vi "alarmes.vi"(0 "NXT IN":T1) -> (1 "NXT OUT":T1, 2 "FinalizarPrograma?":bool)   [LabVIEW 2015, in "ExemploFinal.lvrbt"]
uses:
  ExemploFinal.lvrbt
  <vilib>/NXT/Subs/LVHSConnector.ctl
  <vilib>/NXT/LegoClasses/BrickReference/BrickReference.lvclass
  <vilib>/NXT/Dual Mode Library/Waits/Wait_Num.vi
  <vilib>/NXT/Dual Mode Library/Sound/PlayC.vi
  <vilib>/NXT/Dual Mode Library/Sound/PlayB.vi
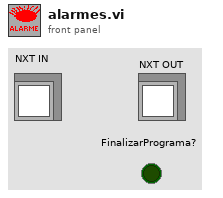
[diagram p1: front panel]
types:
  T1 = typedef "LVHSConnector.ctl" = refnum<class "BrickReference.lvclass">
  T2 = cluster{"TouchOUT":bool, "SomOUT":i32, "LuzOUT":i32, "UltrasomOUT":i32, "BotãoOUT":bool}
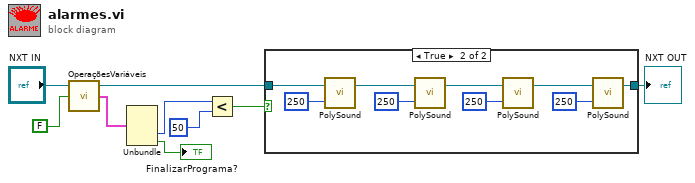
[diagram p0: block diagram]
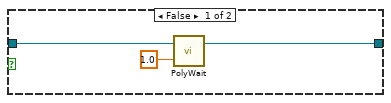
[diagram p2: hidden frame]
diagram:
  n1 = call "OperaçõesVariáveis.vi"("Escrever?"=FALSE, "NXT IN"="NXT IN") -> ("Saídas"=w7:T2, "NXT OUT"=w4:T1)  [unwired: 1 in, 1 out]
  n2 = Unbundle(w7) -> ("UltrasomOUT"=w9:i32, "BotãoOUT"=→"FinalizarPrograma?":bool)  [unwired: 3 out]
  n3 = Less?(x=w9, y=50) -> (x < y?=w2:bool)
  n4 = case shown="True" w2 {
    tunnel: w4 -> [w12 w14]
    tunnel: [w11 w13] -> w6
    frame False {
      n5 = call-poly <vilib>:"PolyWait.vi"("Time (1 sec)"=sgl 1.0, "NXT/EV3"=w12) -> ("NXT/EV3"=w11:T1)  [unwired: 2 in]
    }
    frame True {
      n6 = call-poly <vilib>:"PolySound.vi"("Duration (500 ms)"=u16 250, "NXT/EV3"=w14) -> ("NXT/EV3"=w18:T1)  [unwired: 2 in]
      n7 = call-poly <vilib>:"PolySound.vi"("Duration (500 ms)"=u16 250, "NXT/EV3"=w18) -> ("NXT/EV3"=w15:T1)  [unwired: 2 in]
      n8 = call-poly <vilib>:"PolySound.vi"("Duration (500 ms)"=u16 250, "NXT/EV3"=w15) -> ("NXT/EV3"=w19:T1)  [unwired: 2 in]
      n9 = call-poly <vilib>:"PolySound.vi"("Duration (500 ms)"=u16 250, "NXT/EV3"=w19) -> ("NXT/EV3"=w13:T1)  [unwired: 2 in]
    }
  }
  "NXT OUT" <- w6
